vi "PeltierSafetyTestScript.vi"() -> ()   [LabVIEW 2019]
uses:
  <vilib>/Utility/error.llb/DialogType.ctl
  <vilib>/DAQmx/write.llb/DAQmx Write (Digital Bool 1Line 1Point).vi
  <vilib>/DAQmx/read.llb/DAQmx Read (Analog DBL 1Chan 1Samp).vi
  <vilib>/DAQmx/create/channels.llb/DAQmx Create Channel (DO-Digital Output).vi
  <vilib>/DAQmx/miscellaneous.llb/DAQmx Fill In Error Info.vi
  <instrlib>/BK Precision 178XB Series/BK Precision 178XB Series.lvlib
panel:
  out "Thermocouple 2":dbl
  out "temp. Graph 2":dbl(graph)
  out "Waveform Chart 2":dbl[](graph)
  out "error out":errorcluster
  in  "Current Limit (3 A)":dbl min=0.0 max=6.0 format="%#.2g"
  in  "Maximum Output Voltage (18)":dbl=18.0 min=0.0 max=72.0 format="%#.2f"
  in  "VISA resource name":refnum<visa-resource-name>
  in  "file (use dialog)":path=path "C:/Users/Aniket/Desktop/mCherry_calibration/new_lens/laser_calibration/laser_input.txt"
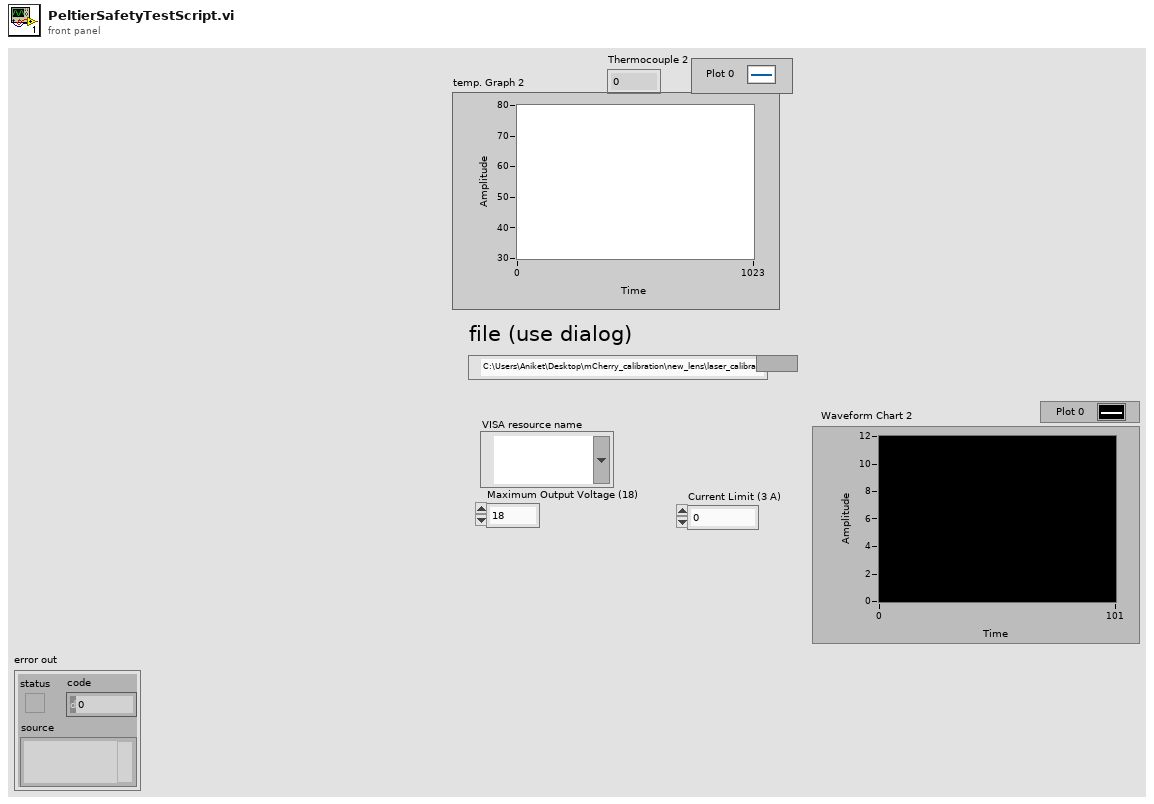
[diagram p1: front panel]
types:
  T1 = typedef "DialogType.ctl" = u16
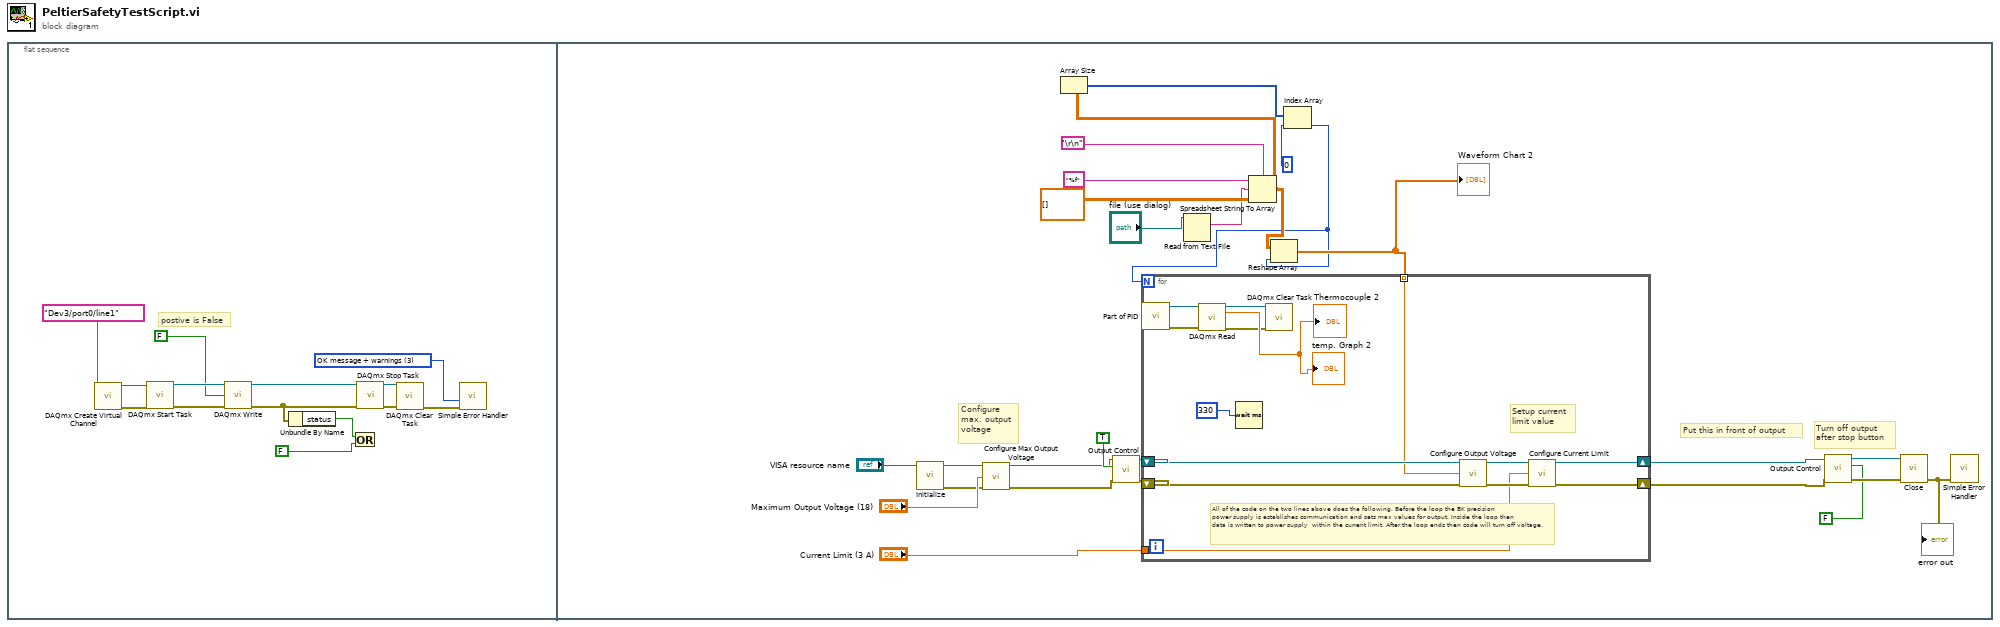
[diagram p0: block diagram]
diagram:
  n1 = flat-sequence {
    frame #0 {
      w14 = T1 3 items=["no dialog", "OK message", "continue or stop message", "OK message + warnings", "continue/stop + warnings"] ("type of dialog (OK msg:1)")
      # "postive is False"
      n2 = call-poly <vilib>:"DAQmx Create Virtual Channel.vi"("lines"=tag "Dev3/port0/line1" ("Line(s)")) -> ("task out"=w9:refnum<k21>, "error out"=w8:errorcluster)  [unwired: 13 in]
      n3 = call <vilib>:"DAQmx Start Task.vi"("task/channels in"=w9, "error in"=w8) -> ("task out"=w4:refnum<k21>, "error out"=w5:errorcluster)  [unwired: 12 in]
      n4 = call-poly <vilib>:"DAQmx Write.vi"("task/channels in"=w4, "data"=FALSE ("Reverse Polarity"), "error in"=w5) -> ("task out"=w12:refnum<k21>, "error out"=w13:errorcluster)  [unwired: 10 in, 1 out]
      n5 = Unbundle By Name(w13) -> ("status"=w3:bool)
      n6 = Or(x=w3, y=FALSE ("Stop")) -> ()  [unwired: 1 out]
      n7 = call <vilib>:"DAQmx Stop Task.vi"("task/channels in"=w12, "error in"=w13) -> ("task out"=w10:refnum<k21>, "error out"=w11:errorcluster)  [unwired: 12 in]
      n8 = call <vilib>:"DAQmx Clear Task.vi"("task in"=w10, "error in"=w11) -> ("error out"=w6:errorcluster)  [unwired: 13 in]
      n9 = call <vilib>:"Simple Error Handler.vi"("type of dialog (OK msg:1)"=w14, "error in (no error)"=w6) -> ()  [unwired: 3 in, 5 out]
    }
    frame #1 {
      # "Put this in front of output"
      # "Turn off output\nafter stop button"
      # "Configure\nmax. output\nvoltage"
      n10 = call "Initialize.vi"("VISA resource name"="VISA resource name") -> ("error out"=w37:errorcluster, "VISA resource name out"=w38:refnum<visa-resource-name>)  [unwired: 9 in]
      n11 = call "Configure Max Output Voltage.vi"("VISA resource name"=w38, "Maximum Output Voltage (18)"="Maximum Output Voltage (18)", "error in (no error)"=w37) -> ("VISA resource name out"=w15:refnum<visa-resource-name>, "error out"=w16:errorcluster)  [unwired: 11 in]
      n12 = call "Output Control.vi"("error in (no error)"=w16, "Enable Output Terminals (F: Off)"=TRUE, "VISA resource name"=w15) -> ("error out"=w25:errorcluster, "VISA resource name out"=w24:refnum<visa-resource-name>)  [unwired: 7 in]
      n13 = Read from Text File(file (use dialog)="file (use dialog)") -> (text=w21:string)  [unwired: 3 in, 3 out]
      n14 = Spreadsheet String To Array(delimiter (Tab)="\r\n", format string="%f", spreadsheet string=w21, array type (2D Dbl)=dbl[][] []) -> (array=w32:dbl[][])
      n15 = Array Size(array=w32) -> (size(s)=w31:i32[])
      n16 = Index Array(array=w31, index=0) -> (element=w20:i32)
      n17 = Reshape Array(w32, w20) -> (w23:dbl[])
      "Waveform Chart 2" <- w23
      n18 = for {
        N: w20 -> [_]
        shift-right: [w48] -> w19
        shift-left: w24 -> [w52]
        shift-right: [w47] -> w18
        shift-left: w25 -> [w51]
        tunnel: w23 -> [w50] mode=indexing
        tunnel: "Current Limit (3 A)" -> [w41]
        # "All of the code on the two lines above does the following. Before the loop the BK precision \npower supply is establishes communication and sets max values for output. Inside the loop then \ndata is written to power supply  within the current limit. After the loop ends then code will turn off voltage."
        # "Setup current\nlimit value"
        n19 = call "Part of PID.vi"() -> ("error out"=w43:errorcluster, "task out"=w42:refnum<k21>)  [unwired: 10 in]
        n20 = call-poly <vilib>:"DAQmx Read.vi"("task/channels in"=w42, "error in"=w43) -> ("task out"=w45:refnum<k21>, "data"=→"temp. Graph 2" →"Thermocouple 2":dbl, "error out"=w44:errorcluster)  [unwired: 11 in]
        n21 = Wait (ms)(milliseconds to wait=u32 330 ("millisecond timer value")) -> ()  [unwired: 1 out]
        n22 = call <vilib>:"DAQmx Clear Task.vi"("task in"=w45, "error in"=w44) -> ()  [unwired: 13 in, 1 out]
        n23 = call "Configure Output Voltage.vi"("VISA resource name"=w52, "Output Voltage (0)"=w50, "error in (no error)"=w51) -> ("VISA resource name out"=w54:refnum<visa-resource-name>, "error out"=w53:errorcluster)  [unwired: 11 in]
        n24 = call "Configure Current Limit.vi"("VISA resource name"=w54, "Current Limit (0)"=w41, "error in (no error)"=w53) -> ("VISA resource name out"=w48:refnum<visa-resource-name>, "error out"=w47:errorcluster)  [unwired: 11 in]
      }
      n25 = call "Output Control.vi"("error in (no error)"=w18, "Enable Output Terminals (F: Off)"=FALSE, "VISA resource name"=w19) -> ("error out"=w34:errorcluster, "VISA resource name out"=w35:refnum<visa-resource-name>)  [unwired: 7 in]
      n26 = call "Close.vi"("error in (no error)"=w34, "VISA resource name"=w35) -> ("error out"=w36:errorcluster)  [unwired: 9 in]
      "error out" <- w36
      n27 = call <vilib>:"Simple Error Handler.vi"("error in (no error)"=w36) -> ()  [unwired: 4 in, 5 out]
    }
  }
